vi "parse1dOr2dArray.vi"(8 "error in (no error)":errorcluster, 10 "<JSON>":string, 11 "$Path or Item Name":string) -> (0 "error out":errorcluster, 3 "Data":dbl[][](array[numeric]))   [LabVIEW 2020, in "horiba.lvlib" / "CCD.lvclass"]
doc: "Parse json arrays into LV arrays."
uses:
  CCD.lvclass
  4735fa6f-9003-4051-a443-cf6d84309e1c.vi
  21661c51-9693-4c48-bb75-1a42afbc6336.vi
  <vilib>/JDP Science/JSONtext/Find Item.vi
  <vilib>/JDP Science/JSONtext/Next JSON Value.vi
  <vilib>/JDP Science/JSONtext/String Subset.vi
  <vilib>/JDP Science/JSONtext/Parsing/Advance past next JSON Value (inlined COPY).vi
  <vilib>/JDP Science/JSONtext/Parsing/Advance past whitespace.vi
  <vilib>/JDP Science/JSONtext/Parsing/Advance past String.vi
  <vilib>/JDP Science/JSONtext/Parsing/Advance past Number.vi
  <vilib>/JDP Science/JSONtext/Parsing/Advance past Line Ending.vi
  <vilib>/JDP Science/JSONtext/Parsing/Parse Full Path or Item Name.vi
  <vilib>/JDP Science/JSONtext/Parsing/Advance past Array.vi
  <vilib>/JDP Science/JSONtext/Parsing/Advance past Object.vi
  <vilib>/JDP Science/JSONtext/support/Error Cluster From Code.vi
  <vilib>/JDP Science/JSONtext/Offset/Find Item Locations by Path.vi
  <vilib>/JDP Science/JSONtext/JSON text to Variant.vi
  <vilib>/JDP Science/JSONtext/LVClass Serializer/JSONtext LVClass Serializer.lvclass
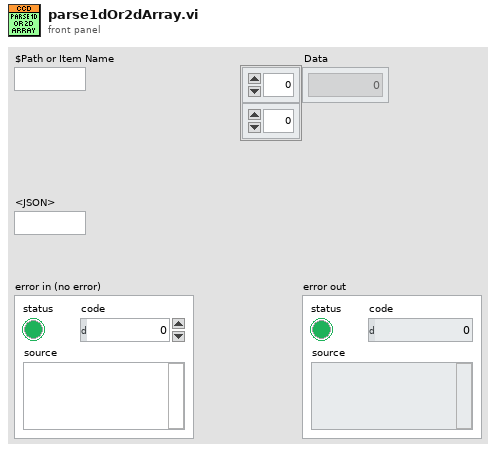
[diagram p1: front panel]
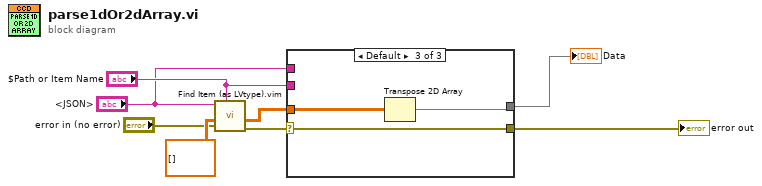
[diagram p0: block diagram]
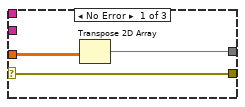
[diagram p2: hidden frame]
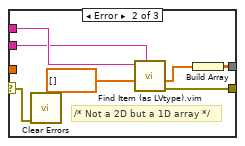
[diagram p3: hidden frame]
diagram:
  n1 = call "Find Item (as LVtype).vim"("$Path or Item Name"="$Path or Item Name", "error in (no error)"="error in (no error)", "Data Type and Default Value"=dbl[][] [] ("xyData"), "JSON"="<JSON>") -> ("error out"=w3:errorcluster, "Data"=w4:dbl[][])  [unwired: 4 in, 2 out]
  n2 = case shown="Default" w3 {
    selector: w3 -> [w9 w18 w20]
    tunnel: w4 -> [w10 _ w21]
    tunnel: [w11 w13 w19] -> w5
    tunnel: [w9 w15 w20] -> w6
    tunnel: "<JSON>" -> [_ w16 _]
    tunnel: "$Path or Item Name" -> [_ w12 _]
    frame No Error {
      n3 = Transpose 2D Array(2D array=w10) -> (transposed array=w11:dbl[][])
    }
    frame Error {
      # "/* Not a 2D but a 1D array */"
      n4 = call <vilib>:"Clear Errors.vi"("error in (no error)"=w18) -> ()  [unwired: 5 in, 2 out]
      n5 = call "Find Item (as LVtype).vim"("$Path or Item Name"=w12, "Data Type and Default Value"=dbl[] [] ("xyData"), "JSON"=w16) -> ("error out"=w15:errorcluster, "Data"=w14:dbl[])  [unwired: 5 in, 2 out]
      n6 = Build Array(w14) -> (w13:dbl[][])
    }
    frame Default {
      n7 = Transpose 2D Array(2D array=w21) -> (transposed array=w19:dbl[][])
    }
  }
  "error out" <- w6
  "Data" <- w5
